vi "Wrapper_setIntegrationTime_Mod.vi"(8 "error in (no error)":errorcluster caption="entrée d'erreur (pas d'erreur)", 9 "Integration Time":i32, 10 "Wrapper In":u32, 11 "Index":i32) -> (0 "error out":errorcluster caption="sortie d'erreur", 2 "Wrapper Out":u32)   [LabVIEW 2024]
uses:
  OmniDriver32.dll
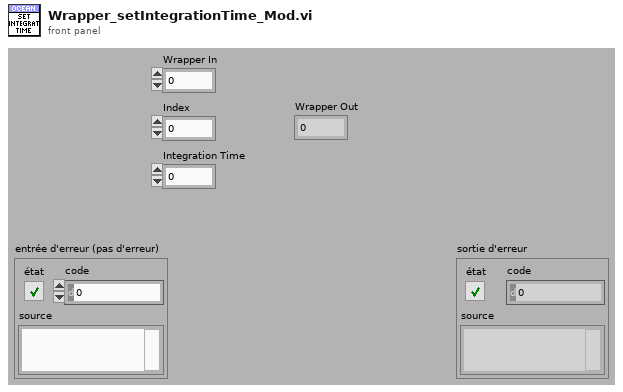
[diagram p1: front panel]
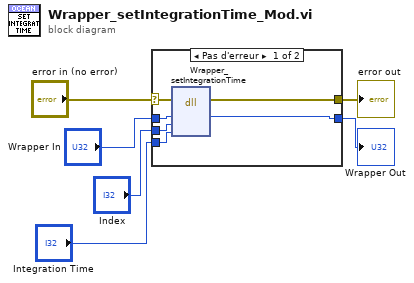
[diagram p0: block diagram]
diagram:
  n1 = case shown="Pas d'erreur" "error in (no error)" {
    selector: "error in (no error)" -> [w7 w14]
    tunnel: "Wrapper In" -> [w12 w13]
    tunnel: "Index" -> [w11 _]
    tunnel: "Integration Time" -> [w10 _]
    tunnel: [w9 w13] -> w3
    tunnel: [w8 w14] -> w2
    frame No Error {
      n2 = dll-call lib="OmniDriver32.dll" fn="Wrapper_setIntegrationTime" label="Wrapper.setIntegrationTime"(error in=w7, "Wrapper"=w12, "Index"=w11, "Integration Time"=w10) -> (error out=w8:errorcluster, "Wrapper"=w9:u32)  [unwired: 4 in, 2 out]
    }
    frame Error {
    }
  }
  "Wrapper Out" <- w3
  "error out" <- w2
